vi "TestCodeOut.vi"() -> ()   [LabVIEW 2018]
doc: "VI used to test different portions of code before they are incorporated into the main code."
uses:
  <vilib>/Utility/error.llb/Error Cluster From Error Code.vi
  <vilib>/ErrorRing/Error Ring.xnode
  NistPluggableModules/TestClass/Test.lvclass
panel:
  in  "Error In":errorcluster
  out "Error":errorcluster
  out "ModuleIndex":i32
  in  "ModuleType":string
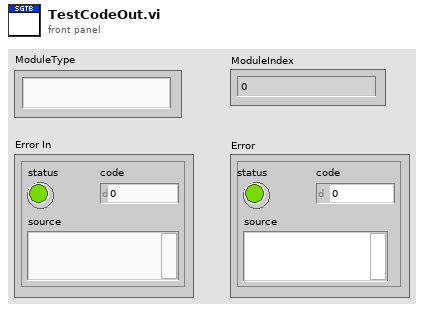
[diagram p1: front panel]
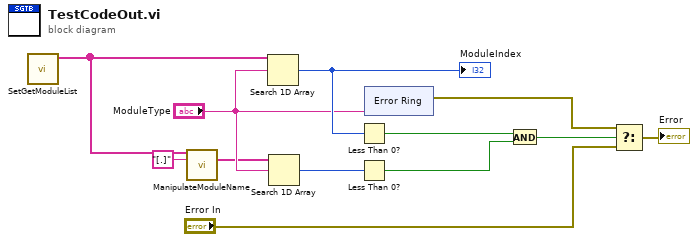
[diagram p0: block diagram]
diagram:
  n1 = call "SetGetModuleList.vi"() -> ("ModuleList"=w3:string[])  [unwired: 11 in]
  n2 = call "ManipulateModuleName.vi"("ModuleListArrayIn"=w3, "MatchExpression"="[.]") -> ("BeforeMatch:ModuleListArray"=w1:string[])  [unwired: 8 in, 5 out]
  n3 = Search 1D Array(1D array=w3, element="ModuleType") -> (index of element=w12:i32)  [unwired: 1 in]
  "ModuleIndex" <- w12
  n4 = Search 1D Array(1D array=w1, element="ModuleType") -> (index of element=w5:i32)  [unwired: 1 in]
  n5 = Less Than 0?(x=w12) -> (x < 0?=w8:bool)
  n6 = Less Than 0?(x=w5) -> (x < 0?=w4:bool)
  n7 = xnode "Error Ring"("parameter 0"="ModuleType") -> ("error out"=w11:errorcluster)
  n8 = And(x=w8, y=w4) -> (x .and. y?=w7:bool)
  n9 = Select(t=w11, s=w7, f="Error In") -> (s? t:f=→"Error":errorcluster)
